vi "unnecessary_multiplication.vi"(1 "N":dbl, 2 "AcqTime ms":dbl) -> (0 "AcqTime Total (s)":dbl)   [LabVIEW 2019]
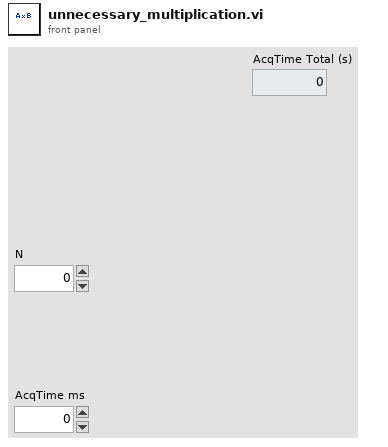
[diagram p1: front panel]
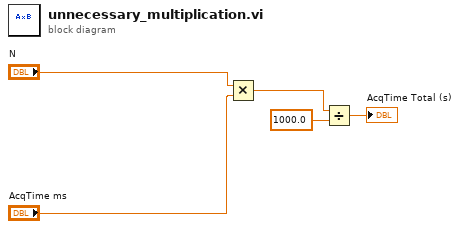
[diagram p0: block diagram]
diagram:
  n1 = Multiply(x="N", y="AcqTime ms") -> (x*y=w3:dbl)
  n2 = Divide(x=w3, y=1000.0) -> (x/y=→"AcqTime Total (s)":dbl)
